vi "CoboltLaser_OutputPowerSet.vi"(0 "ComPort":refnum<visa-resource-name>, 1 "OutputPower (W)":dbl format="%.4g", 3 "CheckResponse":bool=TRUE, 7 "ErrorIn":errorcluster) -> (20 "ComPortOut":refnum<visa-resource-name>, 27 "ErrorOut":errorcluster)   [LabVIEW 2019]
doc: "Use this template to build a VI to use as a subVI."
panel:
  out "ResponseOK":bool
  out "Response":string
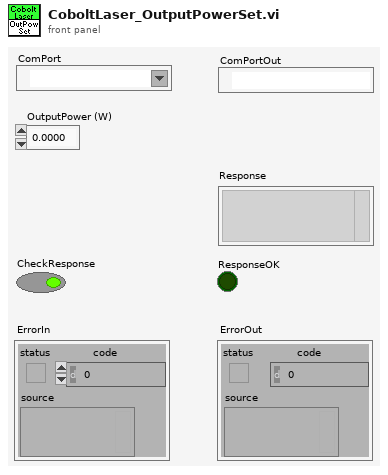
[diagram p1: front panel]
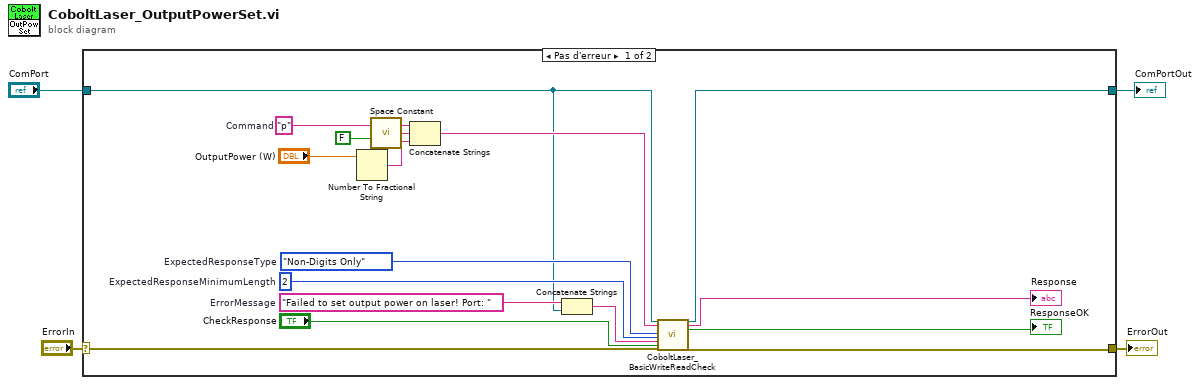
[diagram p0: block diagram]
diagram:
  n1 = case shown="Pas d'erreur" "ErrorIn" {
    selector: "ErrorIn" -> [w21 w23]
    tunnel: [w20 w23] -> w3
    tunnel: "ComPort" -> [w7 w22]
    tunnel: [w6 w22] -> w1
    frame No Error {
      w18 = 2  # ExpectedResponseMinimumLength
      w19 = enum16{"Any", "Digits Only", "Non-Digits Only"}."Non-Digits Only"  # ExpectedResponseType
      w14 = "Failed to set output power on laser! Port: "  # ErrorMessage
      w12 = "p"  # Command
      n2 = Number To Fractional String(use system decimal point (T)=FALSE, number="OutputPower (W)") -> (F-format string=w9:string)  [unwired: 2 in]
      n3 = call <vilib>:"Space Constant.vi"() -> ("String"=w11:string)
      n4 = Concatenate Strings(w12, w11, w9) -> (w8:string)
      n5 = Concatenate Strings(w14, w7) -> (w13:string)
      n6 = call <userlib>:"CoboltLaser_BasicWriteReadCheck.vi"("ComPort"=w7, "Command"=w8, "ExpectedResponseType"=w19, "ExpectedResponseMinimumLength"=w18, "ErrorMessage"=w13, "GenerateError"="CheckResponse", "error in (no error)"=w21) -> ("ComPortOut"=w6:refnum<visa-resource-name>, "Response"=→"Response":string, "ResponseOK"=→"ResponseOK":bool, "error out"=w20:errorcluster)  [unwired: 17 in]
    }
    frame Error {
    }
  }
  "ErrorOut" <- w3
  "ComPortOut" <- w1
